vi "FaultState.vi"(8 "error in (no error)":errorcluster, 11 "Actual Start [i]":i64) -> (0 "error out":errorcluster, 2 "Cluster":T1, 3 "Numeric":i64)   [LabVIEW 2018]
uses:
  Type_Def Actuator Controls.ctl
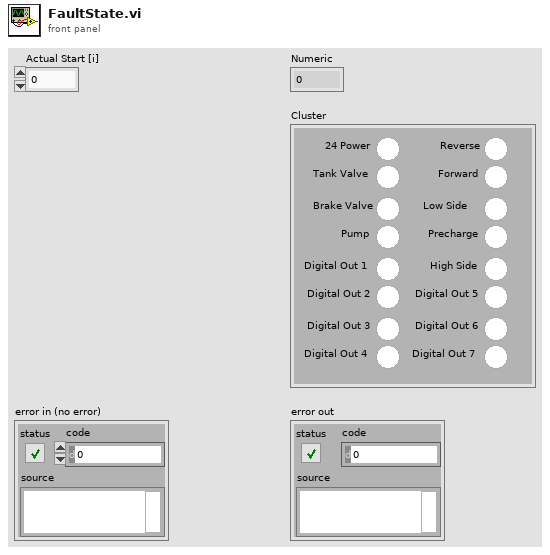
[diagram p1: front panel]
types:
  T1 = typedef "Type_Def Actuator Controls.ctl" = cluster{"Reverse ":bool, "Forward":bool, "Low Side":bool, "Precharge":bool, "High Side":bool, "Digital Out 5":bool, "Digital Out 6":bool, "Digital Out 7 ":bool, "24 Power":bool, "Tank Valve ":bool, "Brake Valve":bool, "Pump":bool, "Digital Out 1 ":bool, "Digital Out 2":bool, "Digital Out 3":bool, "Digital Out 4 ":bool}
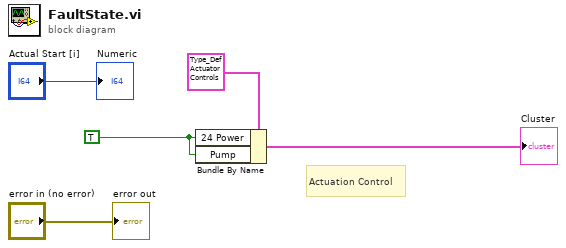
[diagram p0: block diagram]
diagram:
  w3 = TRUE
  # "Actuation Control"
  n1 = Bundle By Name(cluster=T1 {"Reverse "=FALSE, "Forward"=FALSE, "Low Side"=FALSE, "Precharge"=FALSE, "High Side"=FALSE, "Digital Out 5"=FALSE, "Digital Out 6"=FALSE, "Digital Out 7 "=FALSE, "24 Power"=FALSE, "Tank Valve "=FALSE, "Brake Valve"=FALSE, "Pump"=FALSE, "Digital Out 1 "=FALSE, "Digital Out 2"=FALSE, "Digital Out 3"=FALSE, "Digital Out 4 "=FALSE} ("Cluster in 2"), "24 Power"=w3, "Pump"=w3) -> (→"Cluster":T1)
  "error out" <- "error in (no error)"
  "Numeric" <- "Actual Start [i]"
